vi "Event Handle Loop_Mouse Move.vi"(8 "error in (no error)":errorcluster, 10 "Coords":T1, 11 "QMenu Class in":refnum<class "QMenu Class.lvclass">) -> (0 "error out":errorcluster, 3 "QMenu Class out":refnum<class "QMenu Class.lvclass">)   [LabVIEW 2020, in "QTab.lvlib" / "QMenu Class.lvclass"]
uses:
  QMenu Class.lvclass
  <vilib>/Utility/miscctls.llb/LVPoint32TypeDef.ctl
  QMenu Class.lvclass/QMenu Class.ctl
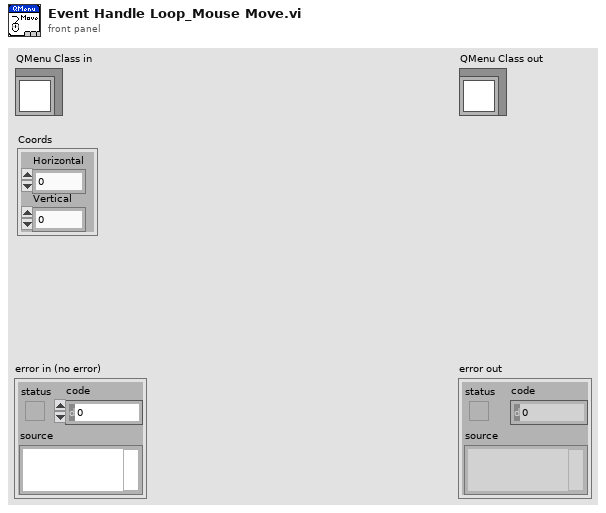
[diagram p1: front panel]
types:
  T1 = typedef "LVPoint32TypeDef.ctl" = cluster{"Horizontal":i32, "Vertical":i32}
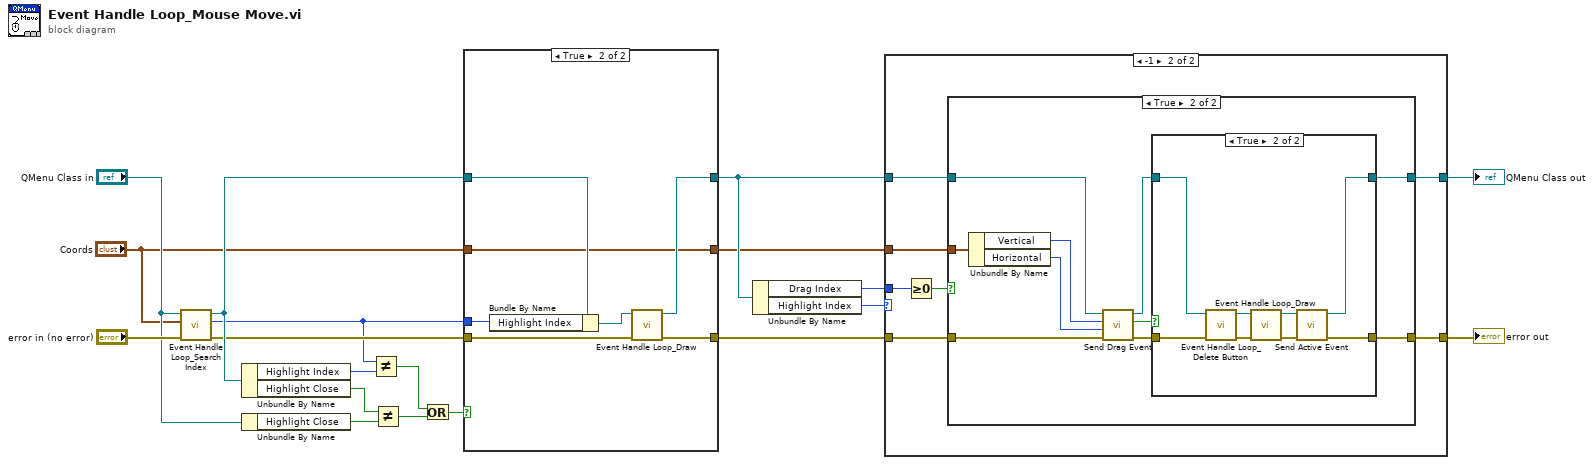
[diagram p0: block diagram]
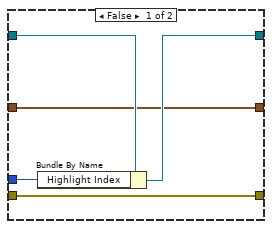
[diagram p5: hidden frame]
diagram:
  n1 = call "Event Handle Loop_Search Index.vi"("error in (no error)"="error in (no error)", "Coords"="Coords", "QMenu Class in"="QMenu Class in") -> ("error out"=w10:errorcluster, "Index"=w9:i32, "QMenu Class out"=w11:refnum<class "QMenu Class.lvclass">)  [unwired: 6 in]
  n2 = Unbundle By Name(w11) -> ("Highlight Index"=w18:i32, "Highlight Close"=w15:bool)
  n3 = Unbundle By Name("QMenu Class in") -> ("Highlight Close"=w16:bool)
  n4 = Not Equal?(x=w9, y=w18) -> (x != y?=w13:bool)
  n5 = Not Equal?(x=w15, y=w16) -> (x != y?=w14:bool)
  n6 = Or(x=w13, y=w14) -> (x .or. y?=w12:bool)
  n7 = case shown="True" w12 {
    tunnel: w11 -> [w23 w31]
    tunnel: [w21 w27] -> w7
    tunnel: w10 -> [w22 w29]
    tunnel: w9 -> [w24 w30]
    tunnel: [w22 w26] -> w8
    tunnel: "Coords" -> [w20 w25]
    tunnel: [w20 w25] -> w1
    frame False {
      n8 = Bundle By Name(cluster=w23, "Highlight Index"=w24) -> (w21:refnum<class "QMenu Class.lvclass">)
    }
    frame True {
      n9 = Bundle By Name(cluster=w31, "Highlight Index"=w30) -> (w28:refnum<class "QMenu Class.lvclass">)
      n10 = call "Event Handle Loop_Draw.vi"("error in (no error)"=w29, "QMenu Class in"=w28) -> ("error out"=w26:errorcluster, "QMenu Class out"=w27:refnum<class "QMenu Class.lvclass">)  [unwired: 8 in]
    }
  }
  n11 = Unbundle By Name(w7) -> ("Drag Index"=w3:i32, "Highlight Index"=w4:i32)
  n12 = case shown="-1" w4 {
    tunnel: w8 -> [w32 w40]
    tunnel: w7 -> [w33 w39]
    tunnel: [w33 w38] -> w6
    tunnel: [w32 w37] -> w5
    tunnel: w3 -> [_ w36]
    tunnel: w1 -> [_ w34]
    frame Default {
    }
    frame -1 {
      n13 = Greater Or Equal To 0?(x=w36) -> (x >= 0?=w35:bool)
      n14 = case shown="True" w35 {
        tunnel: w40 -> [w41 w52]
        tunnel: w39 -> [w42 w51]
        tunnel: [w42 w43] -> w38
        tunnel: [w41 w44] -> w37
        tunnel: w34 -> [_ w50]
        frame False {
        }
        frame True {
          n15 = Unbundle By Name(w50) -> ("Vertical"=w48:i32, "Horizontal"=w49:i32)
          n16 = call "Send Drag Event.vi"("error in (no error)"=w52, "Horizontal"=w49, "Vertical"=w48, "QMenu Class in"=w51) -> ("error out"=w47:errorcluster, "Confirm"=w46:bool, "QMenu Class out"=w45:refnum<class "QMenu Class.lvclass">)  [unwired: 5 in]
          n17 = case shown="True" w46 {
            tunnel: w47 -> [w53 w58]
            tunnel: w45 -> [w54 w57]
            tunnel: [w53 w56] -> w44
            tunnel: [w54 w55] -> w43
            frame False {
            }
            frame True {
              n18 = call "Event Handle Loop_Delete Button.vi"("error in (no error)"=w58, "QMenu Class in"=w57) -> ("error out"=w59:errorcluster, "QMenu Class out"=w60:refnum<class "QMenu Class.lvclass">)  [unwired: 8 in]
              n19 = call "Event Handle Loop_Draw.vi"("error in (no error)"=w59, "QMenu Class in"=w60) -> ("error out"=w62:errorcluster, "QMenu Class out"=w61:refnum<class "QMenu Class.lvclass">)  [unwired: 8 in]
              n20 = call "Send Active Event.vi"("error in (no error)"=w62, "QMenu Class in"=w61) -> ("error out"=w56:errorcluster, "QMenu Class out"=w55:refnum<class "QMenu Class.lvclass">)  [unwired: 8 in]
            }
          }
        }
      }
    }
  }
  "error out" <- w5
  "QMenu Class out" <- w6
